vi "IPS Set Target Field.vi"(3 "Error In":errorcluster={"status"=FALSE, "code"=1073676294, "source"="VISA Read in Prologix USB GPIB Command.vi"}, 4 "Target Field (T)":dbl=0.025, 5 "VISA resource name":refnum<visa-resource-name>="GPIB1::25::INSTR") -> (0 "Error Out":errorcluster={"status"=TRUE, "code"=-1073807346, "source"="VISA Open in NI USB GPIB Command.vi->IPS Set Target Field.vi->IV_B_2Gates_4461-4462.vi"}, 1 "Output":string, 2 "VISA resource name":refnum<visa-resource-name>)   [LabVIEW 2013]
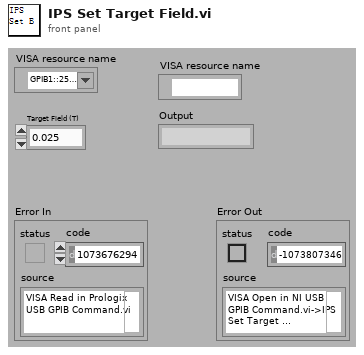
[diagram p1: front panel]
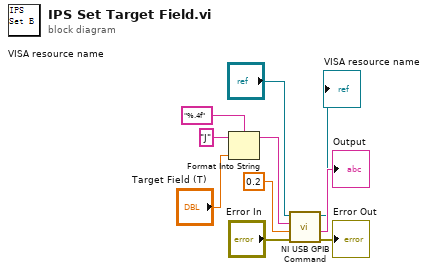
[diagram p0: block diagram]
diagram:
  n1 = Format Into String(format string="%.4f", initial string="J" ("string (\"\")"), "Target Field (T)") -> (resulting string=w2:string)  [unwired: 1 in, 1 out]
  n2 = call "NI USB GPIB Command.vi"("Error In"="Error In", "Wait for instrument to respond (s)"=0.2, "String to Send"=w2, "VISA resource name (COM Port of Prologix Device)"="VISA resource name") -> ("Error Out"=→"Error Out":errorcluster, "Return String from Device (Not all commands return a String)"=→"Output":string, "VISA resource name (COM Port of Prologix Device) 2"=→"VISA resource name":refnum<visa-resource-name>)  [unwired: 1 out]
